vi "Value.vi"(8 "Error In":errorcluster, 11 "Number Widget In":refnum<class "Number Widget.lvclass">) -> (0 "Error Out":errorcluster, 2 "Value":dbl, 3 "Number Widget Out":refnum<class "Number Widget.lvclass">)   [LabVIEW 2014, in "6. Reusing Components Dynamically.lvlib" / "Number Widget.lvclass"]
doc: "Gets the value of the LCD and slider.\n\n\nCopyright (c) 2019 Sze Howe Koh.\nThis code is licensed under the MIT license."
uses:
  Number Widget.lvclass
  Number Widget.lvclass/Number Widget.ctl
  <vilib>/addons/LQ/Qwt/QwtAbstractSlider/QwtAbstractSlider.lvclass
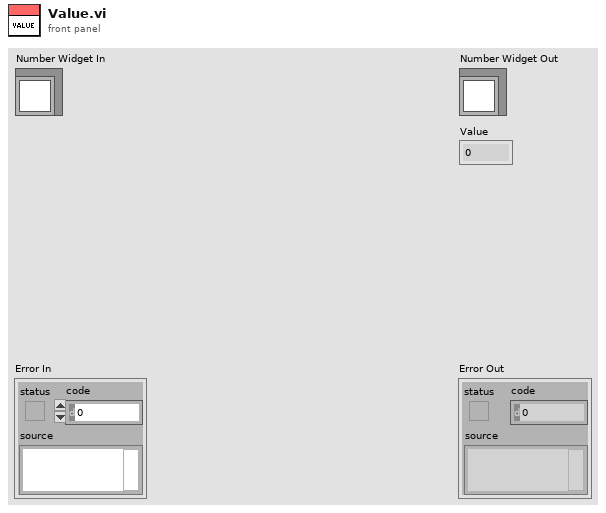
[diagram p1: front panel]
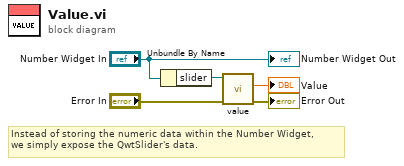
[diagram p0: block diagram]
diagram:
  # "Instead of storing the numeric data within the Number Widget,\nwe simply expose the QwtSlider's data."
  n1 = Unbundle By Name("Number Widget In") -> ("slider"=w4:refnum<class "QwtSlider.lvclass">)
  n2 = call <vilib>:"value.vi"("Error In"="Error In", "QwtAbstractSlider In"=w4) -> ("Error Out"=→"Error Out":errorcluster, "Value"=→"Value":dbl)  [unwired: 7 in, 1 out]
  "Number Widget Out" <- "Number Widget In"
